vi "ReadBin.vi"() -> ()   [LabVIEW 2014]
panel:
  out "Array":sgl[](array[numeric])
  in  "file path (use dialog)":path
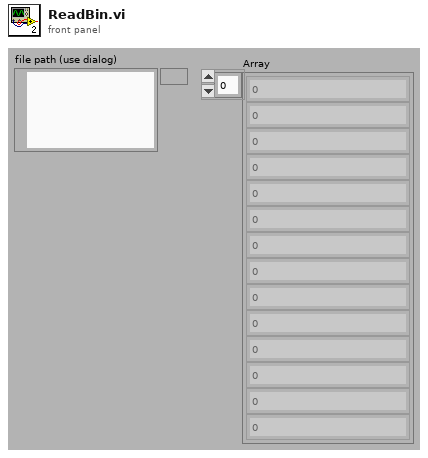
[diagram p1: front panel]
types:
  T1 = enum16{"open", "replace", "create", "open or create", "replace or create", "replace or create with confirmation"}
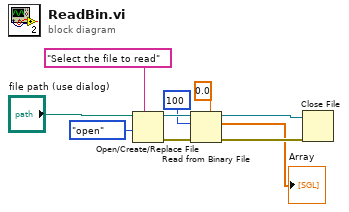
[diagram p0: block diagram]
diagram:
  n1 = Open/Create/Replace File(file path (use dialog)="file path (use dialog)", prompt="Select the file to read", operation (0:open)=T1."open") -> (refnum out=w6:refnum<file>, error out=w7:errorcluster)  [unwired: 3 in, 1 out]
  n2 = Read from Binary File(5:sgl 0.0, 8:w7, 10:100 ("count"), 11:w6) -> (0:w2:errorcluster, 2:→"Array":sgl[], 3:w3:refnum<file>)  [unwired: 2 in, 1 out]
  n3 = Close File(refnum=w3, error in=w2) -> ()  [unwired: 2 out]
